vi "UpdateSerializeWvfm.vi"(7 "LVWSR":refnum<class "Web Request.lvclass">, 11 "page":u8) -> ()   [LabVIEW 2016]
uses:
  <vilib>/wsapi/Web Request.lvclass
  Controller/Messages/Forward Command/Forward Command MSG.lvclass
  C:/Program Files (x86)/National Instruments/LabVIEW 2016/vi.lib/ActorFramework/Message/Message.lvclass
  PAS/Commands/Update Serialize Waveform CMD/Update Serialize Waverform CMD.lvclass
  C:/Program Files (x86)/National Instruments/LabVIEW 2016/vi.lib/MSR Consulting, LLC/General Reuse/Command/Command.lvclass
  PAS/Commands/Update Serialize Waveform CMD/Update Serialize Waverform CMD.lvclass/Update Serialize Waverform CMD.ctl
  Controller/Messages/Forward Command/Forward Command MSG.lvclass/Forward Command MSG.ctl
  <vilib>/ActorFramework/Message Enqueuer/Message Enqueuer.lvclass/Message Enqueuer.ctl
  PAS/Commands/Update Serialize Waveform CMD/Write serialize_.vi
  Controller/Messages/Forward Command/Write id.vi
  Controller/Messages/Forward Command/Write CMD.vi
  <vilib>/ActorFramework/Message Priority Queue/Priority Enqueue.vi
  Controller/gController.lvclass
  <vilib>/ActorFramework/Message Enqueuer/Message Enqueuer.lvclass
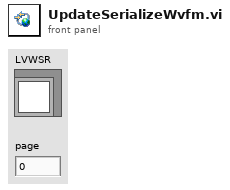
[diagram p1: front panel]
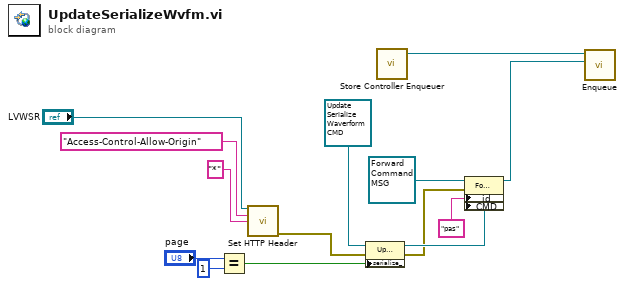
[diagram p0: block diagram]
diagram:
  n1 = Equal?(x="page", y=u8 1) -> (x = y?=w9:bool)
  n2 = call <vilib>:"Set HTTP Header.vi"("LabVIEW Web Service Request"="LVWSR", "header"="Access-Control-Allow-Origin", "header value"="*") -> ("error out"=w4:errorcluster)  [unwired: 11 in, 1 out]
  n3 = property class="Update Serialize Waverform CMD"(reference=refnum<class "Update Serialize Waverform CMD.lvclass"> refnum ("gPAS Library.lvlib:Update Serialize Waverform CMD"), error in=w4, "serialize_"=w9) -> (reference out=w8:refnum<class "Update Serialize Waverform CMD.lvclass">, error out=w3:errorcluster)
  n4 = call "Store Controller Enqueuer.vi"() -> ("Controller Enqueuer Out"=w2:refnum<class "Message Enqueuer.lvclass">)  [unwired: 11 in]
  n5 = property class="Forward Command MSG"(reference=refnum<class "Forward Command MSG.lvclass"> refnum ("Controller.lvlib:Forward Command MSG"), error in=w3, "id"="pas", "CMD"=w8) -> (reference out=w1:refnum<class "Forward Command MSG.lvclass">)  [unwired: 1 out]
  n6 = call <vilib>:"Enqueue.vi"("Message"=w1, "Message Enqueuer in"=w2) -> ()  [unwired: 8 in, 2 out]
